vi "Main.vi"   [LabVIEW 2021]
uses:
  Example/Process/Process/Process.lvclass
  C:/PPLs/LabVIEW-Composed-Actor-Model-LVCAM/LabVIEW-Composed-Actor-Model-LVCAM/LVCAM/LVCAM/LVCAM/LVCAM.lvclass
  LVCAM/LVCAM/Self Actor/Self Actor.lvclass
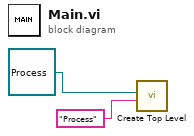
[diagram p0: block diagram]
diagram:
  n1 = call "Create Top Level.vi"("Alias"="Process", "Nest Actor"=refnum<class "Process.lvclass"> refnum ("Process.lvlib:Process.lvclass")) -> ()  [unwired: 10 in]
